vi "RichToFlatgrpc_reflection_v1alpha_ServerReflectionRequest.vi"(5 "OutputClusterType":T1, 11 "InputCluster":T3) -> (3 "OutputCluster":T1)   [LabVIEW 2025, in "reflection_client.lvlib"]
uses:
  reflection_client.lvlib
  grpc_reflection_v1alpha_ServerReflectionRequest.ctl
  grpc_reflection_v1alpha_ServerReflectionRequest_message_request/grpc_reflection_v1alpha_ServerReflectionRequest_message_request.lvclass
  grpc_reflection_v1alpha_ServerReflectionRequest_Flat.ctl
  grpc_reflection_v1alpha_ExtensionRequest_Flat.ctl
  grpc_reflection_v1alpha_ServerReflectionRequest_message_request/grpc_reflection_v1alpha_ServerReflectionRequest_message_request.lvclass/grpc_reflection_v1alpha_ServerReflectionRequest_message_request.ctl
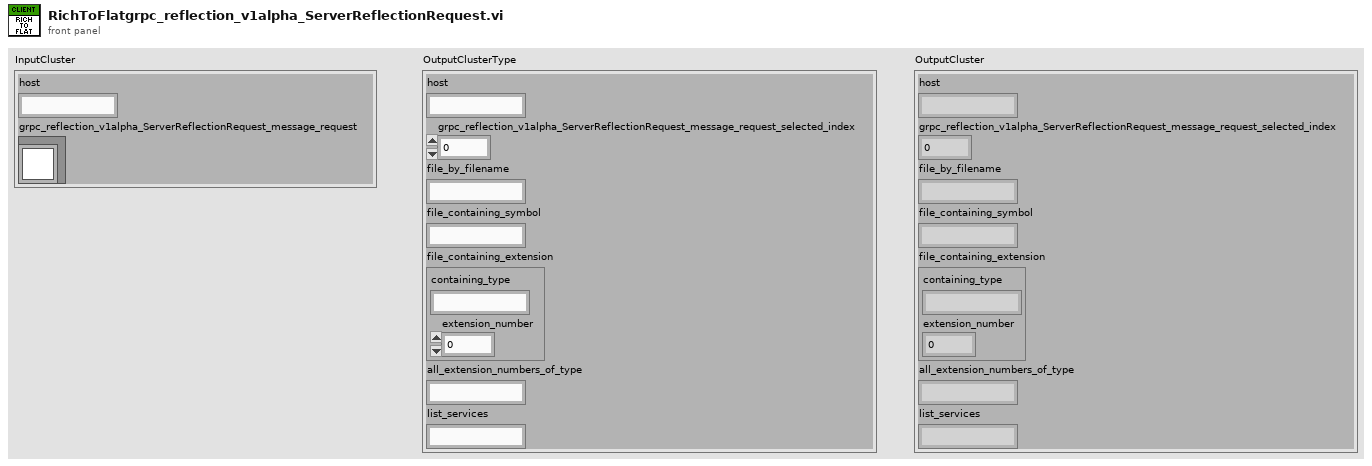
[diagram p1: front panel]
types:
  T1 = typedef "reflection_client.lvlib/grpc_reflection_v1alpha_ServerReflectionRequest_Flat.ctl" = cluster{"host":string, "grpc_reflection_v1alpha_ServerReflectionRequest_message_request_selected_index":i32, "file_by_filename":string, "file_containing_symbol":string, "file_containing_extension":T2, "all_extension_numbers_of_type":string, "list_services":string}
  T2 = typedef "reflection_client.lvlib/grpc_reflection_v1alpha_ExtensionRequest_Flat.ctl" = cluster{"containing_type":string, "extension_number":i32}
  T3 = typedef "reflection_client.lvlib/grpc_reflection_v1alpha_ServerReflectionRequest.ctl" = cluster{"host":string, "grpc_reflection_v1alpha_ServerReflectionRequest_message_request":refnum<class "grpc_reflection_v1alpha_ServerReflectionRequest_message_request.lvclass">}
  T4 = typedef "reflection_client.lvlib/grpc_reflection_v1alpha_ExtensionRequest.ctl" = cluster{"containing_type":string, "extension_number":i32}
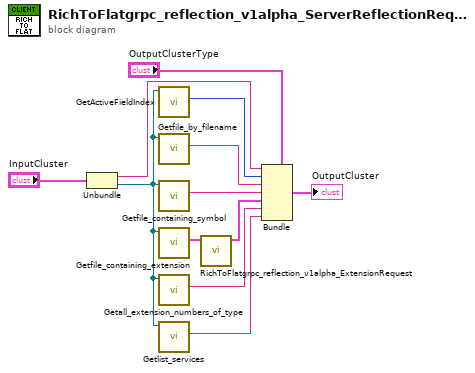
[diagram p0: block diagram]
diagram:
  n1 = Unbundle "Unbundle"("InputCluster") -> ("host"=w9:string, "grpc_reflection_v1alpha_ServerReflectionRequest_message_request"=w8:refnum<class "grpc_reflection_v1alpha_ServerReflectionRequest_message_request.lvclass">)
  n2 = call "GetActiveFieldIndex.vi"("OneOfTemplate in"=w8) -> ("Active Field Index"=w7:i32)  [unwired: 8 in, 2 out]
  n3 = call "Getfile_by_filename.vi"("OneOfTemplate in"=w8) -> ("Get_Val"=w6:string)  [unwired: 8 in, 2 out]
  n4 = call "Getfile_containing_symbol.vi"("OneOfTemplate in"=w8) -> ("Get_Val"=w5:string)  [unwired: 8 in, 2 out]
  n5 = call "Getfile_containing_extension.vi"("OneOfTemplate in"=w8) -> ("Get_Val"=w4:T4)  [unwired: 8 in, 2 out]
  n6 = call "Getall_extension_numbers_of_type.vi"("OneOfTemplate in"=w8) -> ("Get_Val"=w2:string)  [unwired: 8 in, 2 out]
  n7 = call "Getlist_services.vi"("OneOfTemplate in"=w8) -> ("Get_Val"=w1:string)  [unwired: 8 in, 2 out]
  n8 = call "RichToFlatgrpc_reflection_v1alpha_ExtensionRequest.vi"("InputCluster"=w4) -> ("OutputCluster"=w3:T2)  [unwired: 10 in]
  n9 = Bundle "Bundle"(cluster="OutputClusterType", "host"=w9, "grpc_reflection_v1alpha_ServerReflectionRequest_message_request_selected_index"=w7, "file_by_filename"=w6, "file_containing_symbol"=w5, "file_containing_extension"=w3, "all_extension_numbers_of_type"=w2, "list_services"=w1) -> (→"OutputCluster":T1)
